vi "Array of Variants to JSON Object.vi"(4 "LVClass Serializer":refnum<class "JSONtext LVClass Serializer.lvclass">, 5 "enable LabVIEW extensions? (T)":bool=TRUE, 6 "Pretty Print?":bool, 9 "error in (no error)":errorcluster, 10 "Names":string[](array[string]), 11 "Array":variant[](array[variant])) -> (1 "error out":errorcluster, 3 "<JSON>":string caption="<JSON>Object")   [LabVIEW 2017, in "JSONtext.lvlib"]
doc: "Flatten an Array of Variants into a JSON Object. If item names are not supplied, they will be taken from the data name in the Variants.\n\nStrings or Arrays of strings marked with a leading <JSON> tag in their name (including inside clusters) are treated as already being valid JSON. Strings not marked as <JSON> are quoted and escaped as a JSON String."
uses:
  JSONtext.lvlib
  LVClass Serializer/JSONtext LVClass Serializer.lvclass
  <vilib>/Utility/Data Type/NI_Data Type.lvlib
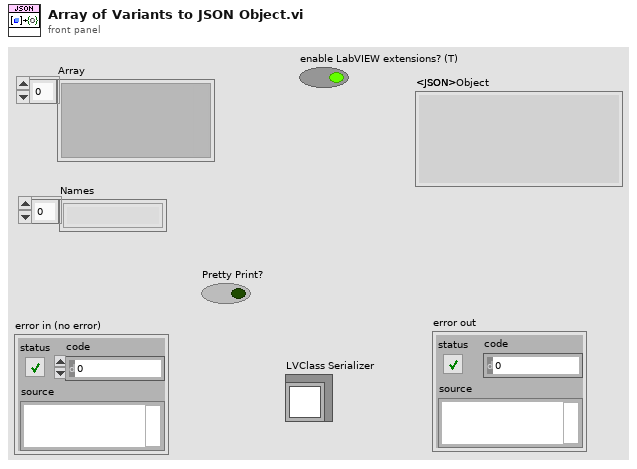
[diagram p1: front panel]
types:
  T1 = typedef "NI_Data Type.lvlib/Data Type.ctl" = enum8{"Invalid Type", "Void", "I8", "I16", "I32", "I64", "U8", "U16", "U32", "U64", "Single Float", "Double Float", "Extended Float", "Single Complex", "Double Complex", "Extended Complex", "Enum U8", "Enum U16", "Enum U32", "Enum U64", "Single Float With Unit", "Double Float With Unit", "Extended Float With Unit", "Single Complex with Unit", "Double Complex with Unit", "Extended Complex with Unit", "Boolean", "String", "Path", "Picture", "Tag", "Array", "Cluster", "Variant", "LV Variant", "Waveform", "Timestamp", "Digital Waveform", "Digital Data", "ExpressData", "Refnum", "External Data", "VI", "Poly VI", "LabVIEW Class Instance", "Fixed Point"}
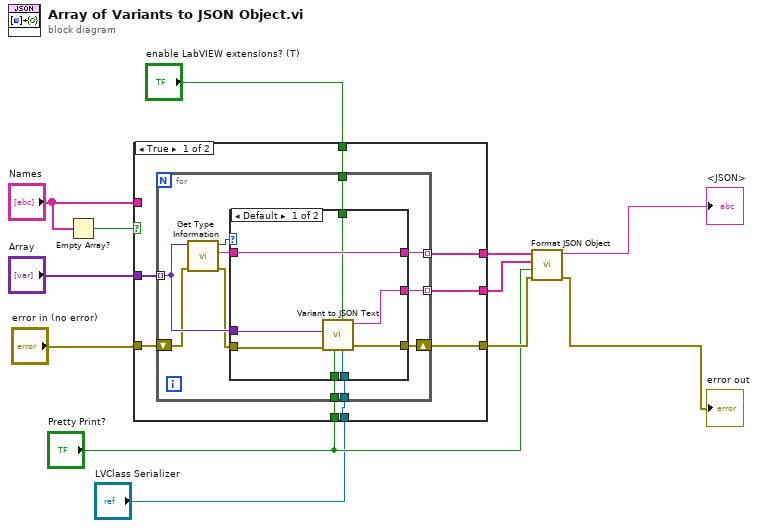
[diagram p0: block diagram]
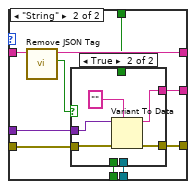
[diagram p2: hidden frame]
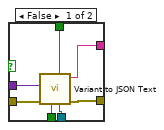
[diagram p3: hidden frame]
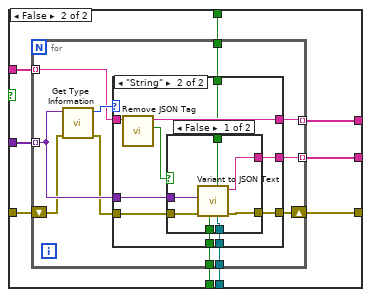
[diagram p4: hidden frame]
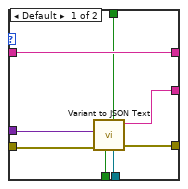
[diagram p5: hidden frame]
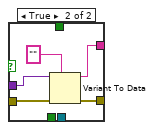
[diagram p6: hidden frame]
diagram:
  n1 = Empty Array?(array="Names") -> (empty?=w5:bool)
  n2 = case shown="True" w5 {
    tunnel: [w20 w70] -> w11
    tunnel: [w19 w69] -> w9
    tunnel: [w18 w68] -> w8
    tunnel: "error in (no error)" -> [w17 w67]
    tunnel: "Array" -> [w16 w66]
    tunnel: "Names" -> [_ w63]
    tunnel: "Pretty Print?" -> [w15 w65]
    tunnel: "enable LabVIEW extensions? (T)" -> [w14 w64]
    tunnel: "LVClass Serializer" -> [w13 w62]
    frame True {
      n3 = for {
        shift-right: [w29] -> w20
        shift-left: w17 -> [w23]
        tunnel: w16 -> [w31] mode=indexing
        tunnel: [w25] -> w19 mode=indexing
        tunnel: [w28] -> w18 mode=indexing
        tunnel: w15 -> [w27]
        tunnel: w14 -> [w26]
        tunnel: w13 -> [w21]
        n4 = call <vilib>:"Get Type Information.vi"("error in (no error)"=w23, "Variant"=w31) -> ("error out"=w22:errorcluster, "Name"=w30:string, "Type"=w24:T1)  [unwired: 5 in, 2 out]
        n5 = case shown="Default" w24 {
          tunnel: w31 -> [w34 w49]
          tunnel: w30 -> [w39 w48]
          tunnel: w22 -> [w35 w47]
          tunnel: [w38 w46] -> w29
          tunnel: [w39 w45] -> w28
          tunnel: w27 -> [w36 w44]
          tunnel: w26 -> [w37 w43]
          tunnel: [w33 w42] -> w25
          tunnel: w21 -> [w32 w40]
          frame Default {
            n6 = call "Variant to JSON Text.vi"("LVClass Serializer"=w32, "enable LabVIEW extensions? (T)"=w37, "Pretty Print?"=w36, "error in (no error)"=w35, "Variant"=w34) -> ("error out"=w38:errorcluster, "<JSON>"=w33:string)  [unwired: 4 in, 1 out]
          }
          frame "String" {
            n7 = call "Remove JSON Tag.vi"("Name"=w48) -> ("tagged as JSON text"=w41:bool, "Name (tag stripped)"=w45:string)  [unwired: 9 in]
            n8 = case shown="True" w41 {
              tunnel: w49 -> [w56 w59]
              tunnel: w47 -> [w55 w60]
              tunnel: [w54 w61] -> w46
              tunnel: w44 -> [w53 _]
              tunnel: w43 -> [w52 _]
              tunnel: [w51 w57] -> w42
              tunnel: w40 -> [w50 _]
              frame False {
                n9 = call "Variant to JSON Text.vi"("LVClass Serializer"=w50, "enable LabVIEW extensions? (T)"=w52, "Pretty Print?"=w53, "error in (no error)"=w55, "Variant"=w56) -> ("error out"=w54:errorcluster, "<JSON>"=w51:string)  [unwired: 4 in, 1 out]
              }
              frame True {
                n10 = Variant To Data(error in=w60, type="", Variant=w59) -> (data=w57:string, error out=w61:errorcluster)
              }
            }
          }
        }
      }
    }
    frame False {
      n11 = for {
        shift-right: [w80] -> w70
        shift-left: w67 -> [w74]
        tunnel: w66 -> [w81] mode=indexing
        tunnel: [w76] -> w69 mode=indexing
        tunnel: [w79] -> w68 mode=indexing
        tunnel: w65 -> [w78]
        tunnel: w64 -> [w77]
        tunnel: w63 -> [w72] mode=indexing
        tunnel: w62 -> [w71]
        n12 = call <vilib>:"Get Type Information.vi"("error in (no error)"=w74, "Variant"=w81) -> ("error out"=w73:errorcluster, "Type"=w75:T1)  [unwired: 5 in, 3 out]
        n13 = case shown="\"String\"" w75 {
          tunnel: w81 -> [w84 w99]
          tunnel: w72 -> [w89 w98]
          tunnel: w73 -> [w85 w97]
          tunnel: [w88 w96] -> w80
          tunnel: [w89 w95] -> w79
          tunnel: w78 -> [w86 w94]
          tunnel: w77 -> [w87 w93]
          tunnel: [w83 w92] -> w76
          tunnel: w71 -> [w82 w90]
          frame Default {
            n14 = call "Variant to JSON Text.vi"("LVClass Serializer"=w82, "enable LabVIEW extensions? (T)"=w87, "Pretty Print?"=w86, "error in (no error)"=w85, "Variant"=w84) -> ("error out"=w88:errorcluster, "<JSON>"=w83:string)  [unwired: 4 in, 1 out]
          }
          frame "String" {
            n15 = call "Remove JSON Tag.vi"("Name"=w98) -> ("tagged as JSON text"=w91:bool, "Name (tag stripped)"=w95:string)  [unwired: 9 in]
            n16 = case shown="False" w91 {
              tunnel: w99 -> [w106 w109]
              tunnel: w97 -> [w105 w110]
              tunnel: [w104 w111] -> w96
              tunnel: w94 -> [w103 _]
              tunnel: w93 -> [w102 _]
              tunnel: [w101 w107] -> w92
              tunnel: w90 -> [w100 _]
              frame False {
                n17 = call "Variant to JSON Text.vi"("LVClass Serializer"=w100, "enable LabVIEW extensions? (T)"=w102, "Pretty Print?"=w103, "error in (no error)"=w105, "Variant"=w106) -> ("error out"=w104:errorcluster, "<JSON>"=w101:string)  [unwired: 4 in, 1 out]
              }
              frame True {
                n18 = Variant To Data(error in=w110, type="", Variant=w109) -> (data=w107:string, error out=w111:errorcluster)
              }
            }
          }
        }
      }
    }
  }
  n19 = call "Format JSON Object.vi"("error in (no error)"=w11, "Pretty Print?"="Pretty Print?", "JSON elements"=w9, "Names"=w8) -> ("error out"=→"error out":errorcluster, "JSON Object Text out"=→"<JSON>":string)  [unwired: 6 in]
